vi "WPI_AccelerometerADXL345_I2C_Get.vi"(8 "error in":errorcluster, 11 "AccelerometerDevRef":T2={"DevStatus"={"status"=FALSE, "code"=0, "source"=""}, "Scaling"={"Gain (VoltsPerG)"=0.0, "Center Voltage"=0.0}, "Analog Channels"={"X-Axis"=enum."Invalid", "Y-Axis"=enum."Invalid", "Z-Axis"=enum."Invalid"}, "I2C Bus"=enum."Invalid", "SPI Bus"=enum."Invalid", "Accel Range"=0, "ADXL Axes"={"X-Axis"=FALSE, "Y-Axis"=FALSE, "Z-Axis"=FALSE}, "Handle"=0, "Device Address"=0, "Accel Type"=enum."Analog"} {"Device Address" format="%.0x"; "Accel Range" items=["+/- 2 g", "+/- 4 g", "+/- 8 g", "+/- 16 g"]}) -> (0 "error out":errorcluster, 2 "Accelerations":T1, 3 "AccelerometerDevRef":T2={"DevStatus"={"status"=FALSE, "code"=0, "source"=""}, "Scaling"={"Gain (VoltsPerG)"=0.0, "Center Voltage"=0.0}, "Analog Channels"={"X-Axis"=enum."Invalid", "Y-Axis"=enum."Invalid", "Z-Axis"=enum."Invalid"}, "I2C Bus"=enum."Invalid", "SPI Bus"=enum."Invalid", "Accel Range"=0, "ADXL Axes"={"X-Axis"=FALSE, "Y-Axis"=FALSE, "Z-Axis"=FALSE}, "Handle"=0, "Device Address"=0, "Accel Type"=enum."Analog"} {"Device Address" format="%.0x"; "Accel Range" items=["+/- 2 g", "+/- 4 g", "+/- 8 g", "+/- 16 g"]})   [LabVIEW 2017]
doc: "Returns the current acceleration of the sensor that you specify.\n\nThis software is licensed. Open the labview\\readme\\WPI Robotics Library Open Source License.txt file for more information."
uses:
  <vilib>/Rock Robotics/WPI/Accelerometer/WPI_AccelerometerDevRef.ctl
  <vilib>/Rock Robotics/WPI/Accelerometer/WPI_AccelerometerScaling.ctl
  <vilib>/Rock Robotics/WPI/Accelerometer/WPI_AccelerometerAnalogChannels.ctl
  <vilib>/Rock Robotics/SystemInterfaces/AI/FPGA_AIChannel.ctl
  <vilib>/Rock Robotics/SystemInterfaces/i2clib/i2c_bus.ctl
  <vilib>/Rock Robotics/SystemInterfaces/spilib/spi_bus.ctl
  <vilib>/Rock Robotics/WPI/Accelerometer/ADXL345 Range.ctl
  <vilib>/Rock Robotics/WPI/Accelerometer/WPI_AccelerometerADXL345 Axes.ctl
  <vilib>/Rock Robotics/WPI/I2C/WPI_I2CDevRef.ctl
panel:
  # "ADXL"
  # "Analog"
  # "ADXL"
  # "Analog"
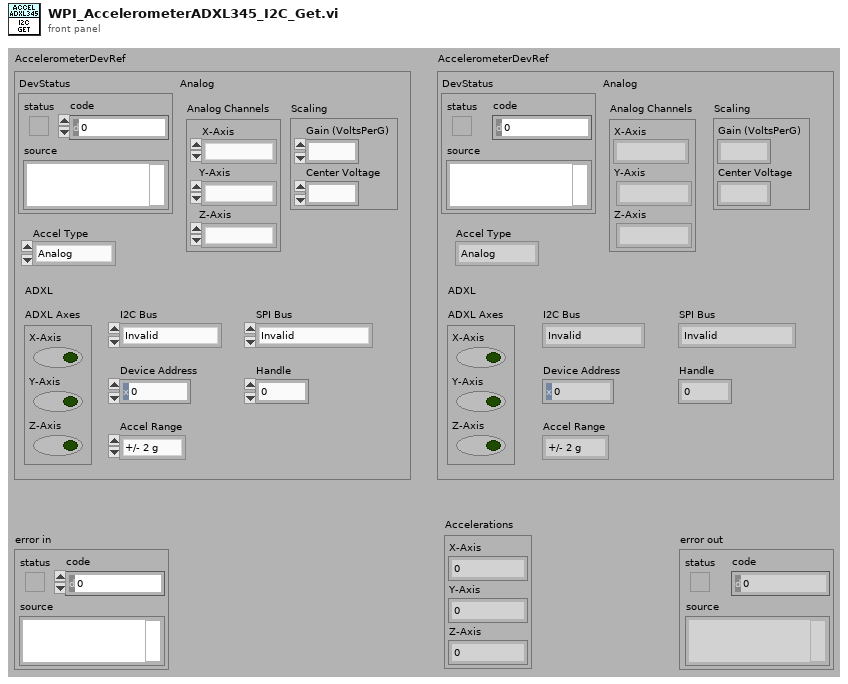
[diagram p1: front panel]
types:
  T1 = cluster{"X-Axis":dbl, "Y-Axis":dbl, "Z-Axis":dbl}
  T2 = typedef "WPI_AccelerometerDevRef.ctl" = cluster{"DevStatus":errorcluster, "Scaling":T3, "Analog Channels":T4, "I2C Bus":T6, "SPI Bus":T7, "Accel Range":T8, "ADXL Axes":T9, "Handle":i32, "Device Address":u8, "Accel Type":enum16{"Analog", "ADXL345 I2C", "ADXL345 SPI", "Internal", "ADXL362 SPI"}}
  T3 = typedef "WPI_AccelerometerScaling.ctl" = cluster{"Gain (VoltsPerG)":dbl, "Center Voltage":dbl}
  T4 = typedef "WPI_AccelerometerAnalogChannels.ctl" = cluster{"X-Axis":T5, "Y-Axis":T5, "Z-Axis":T5}
  T5 = typedef "FPGA_AIChannel.ctl" = enum8{"AI 0", "AI 1", "AI 2", "AI 3", "AI MXP 0", "AI MXP 1", "AI MXP 2", "AI MXP 3", "Invalid"}
  T6 = typedef "i2c_bus.ctl" = enum16{"I2C On-Board", "I2C MXP", "Invalid"}
  T7 = typedef "spi_bus.ctl" = enum16{"SPI On-Board, CS0", "SPI On-Board, CS1", "SPI On-Board, CS2", "SPI On-Board, CS3", "SPI MXP", "Invalid"}
  T8 = typedef "ADXL345 Range.ctl" = u8
  T9 = typedef "WPI_AccelerometerADXL345 Axes.ctl" = cluster{"X-Axis":bool, "Y-Axis":bool, "Z-Axis":bool}
  T10 = typedef "WPI_I2CDevRef.ctl" = cluster{"DevStatus":errorcluster, "Device Address":u8, "Handle":i32, "I2C Bus":T6}
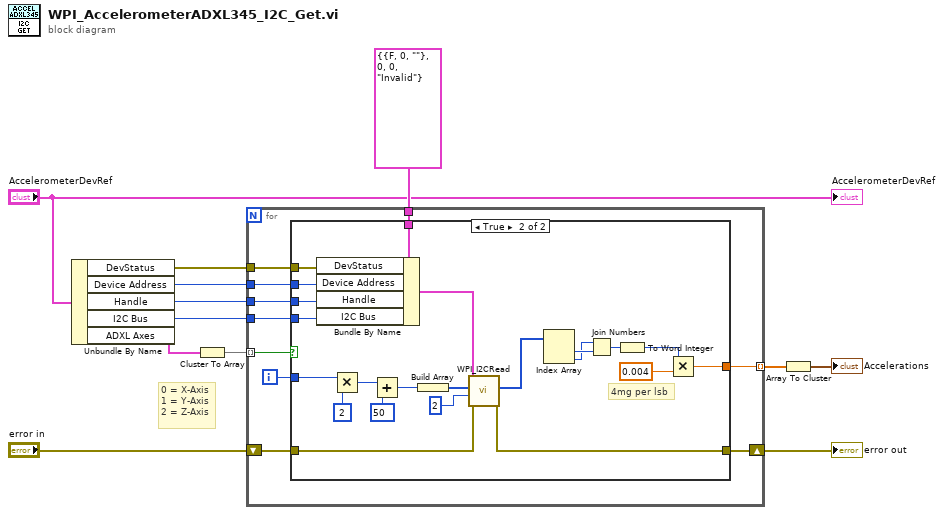
[diagram p0: block diagram]
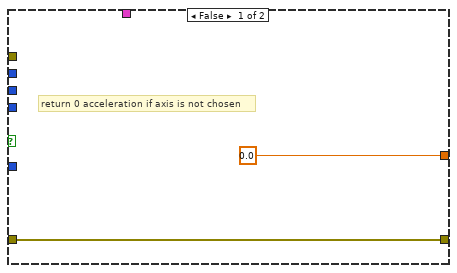
[diagram p2: hidden frame]
diagram:
  # "0 = X-Axis\n1 = Y-Axis\n2 = Z-Axis"
  n1 = Unbundle By Name("AccelerometerDevRef") -> ("DevStatus"=w10:errorcluster, "Device Address"=w4:u8, "Handle"=w8:i32, "I2C Bus"=w7:T6, "ADXL Axes"=w3:T9)
  n2 = Cluster To Array(cluster=w3) -> (array=w2:bool[])
  n3 = for {
    shift-right: [w22] -> w12
    shift-left: "error in" -> [w21]
    tunnel: T10 {"DevStatus"={"status"=FALSE, "code"=0, "source"=""}, "Device Address"=0, "Handle"=0, "I2C Bus"=enum."Invalid"} ("I2CDevRef") -> [w20]
    tunnel: w10 -> [w19]
    tunnel: w8 -> [w18]
    tunnel: w7 -> [w17]
    tunnel: [w16] -> w6 mode=indexing
    tunnel: w4 -> [w15]
    tunnel: w2 -> [w14] mode=indexing
    i -> [w13]
    n4 = case shown="True" w14 {
      tunnel: [w24 w27] -> w22
      tunnel: w21 -> [w24 w28]
      tunnel: w20 -> [_ w46]
      tunnel: w19 -> [_ w45]
      tunnel: w18 -> [_ w32]
      tunnel: w17 -> [_ w31]
      tunnel: [0.0 ("Voltage") w26] -> w16
      tunnel: w15 -> [_ w33]
      tunnel: w13 -> [_ w30]
      frame False {
        # "return 0 acceleration if axis is not chosen"
      }
      frame True {
        # "4mg per lsb"
        n5 = Bundle By Name(cluster=w46, "DevStatus"=w45, "Device Address"=w33, "Handle"=w32, "I2C Bus"=w31) -> (w29:T10)
        n6 = Multiply(x=w30, y=u8 2 ("Data To Send")) -> (x*y=w44:i32)
        n7 = Add(x=w44, y=u8 50 ("Data To Send")) -> (x+y=w36:i32)
        n8 = Build Array(w36) -> (w35:i32[])
        n9 = call <vilib>:"WPI_I2CRead.vi"("error in (no error)"=w28, "I2CBytesToRead"=u8 2, "I2CRegister"=w35, "I2CDevRef"=w29) -> ("error out"=w27:errorcluster, "Data Out"=w40:u8[])  [unwired: 6 out]
        n10 = Index Array(array=w40) -> (element #1=w38:u8, element #2=w37:u8)  [unwired: 2 in]
        n11 = Join Numbers(hi=w37, lo=w38) -> ((hi.lo)=w39:u16)
        n12 = To Word Integer(number=w39) -> (16bit integer=w25:i16)
        n13 = Multiply(x=w25, y=0.004) -> (x*y=w26:dbl)
      }
    }
  }
  "error out" <- w12
  n14 = Array To Cluster(array=w6) -> (cluster=→"Accelerations":cluster{"[0]":dbl, "[1]":dbl, "[2]":dbl})
  "AccelerometerDevRef" <- "AccelerometerDevRef"
